vi "111-by.vi"() -> ()   [LabVIEW 2018]
uses:
  Global_Variable/A131258.vi
panel:
  out "9000-10000分贝最小值":string
  out "9000-10000分贝最大值":string
  out "8000-9000分贝最小值":string
  out "8000-9000分贝最大值":string
  out "7000-8000分贝最小值":string
  out "7000-8000分贝最大值":string
  out "6000-7000分贝最小值":string
  out "6000-7000分贝最大值":string
  out "5000-6000分贝最小值":string
  out "5000-6000分贝最大值":string
  out "4000-5000分贝最小值":string
  out "4000-5000分贝最大值":string
  out "3000-4000分贝最小值":string
  out "3000-4000分贝最大值":string
  out "2000-3000分贝最小值":string
  out "2000-3000分贝最大值":string
  out "数组大小":string
  out "1000-2000分贝最小值":string
  out "1000-2000分贝最大值":string
  out "0-1000分贝最小值":string
  out "0-1000分贝最大值":string
  in  "restart averaging (F)":bool
  out "判定结果":bool
  in  "频率":cluster{"f0":dbl, "df":dbl, "magnitude":dbl[]}[](graph)
  out "加速度":cluster{"f0":dbl, "df":dbl, "magnitude":dbl[]}[](graph)
  # "060芯轴总成NVH评价"
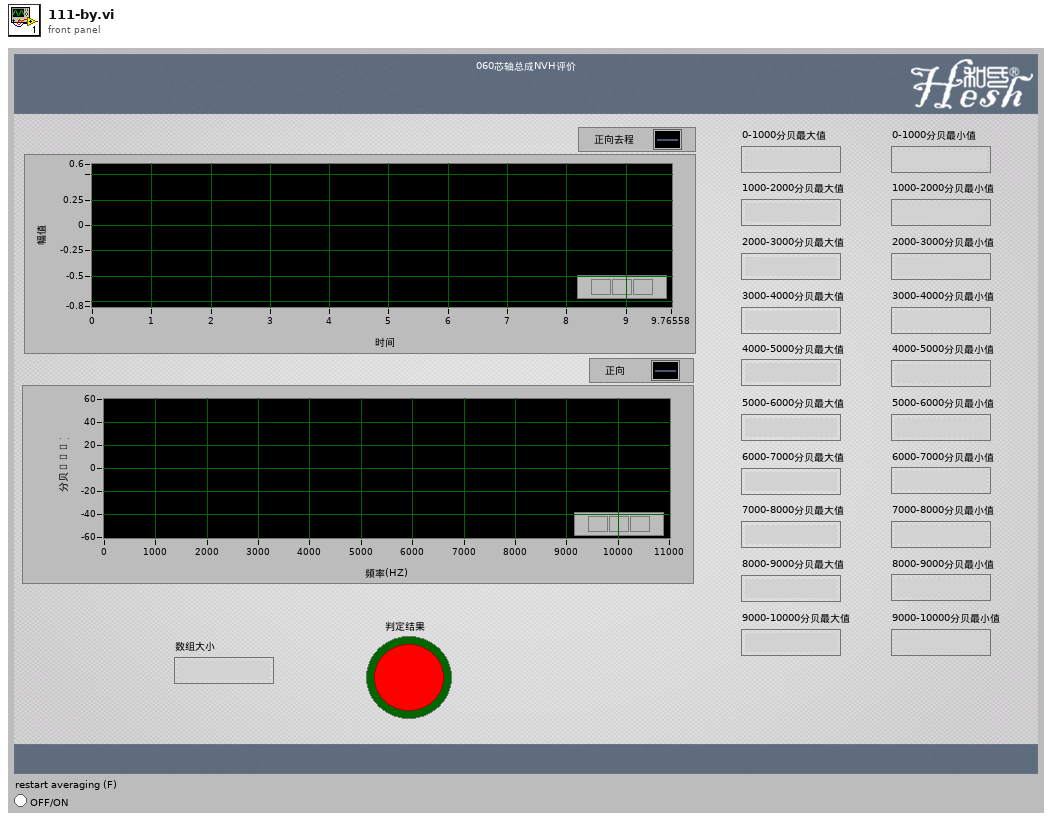
[diagram p1: front panel]
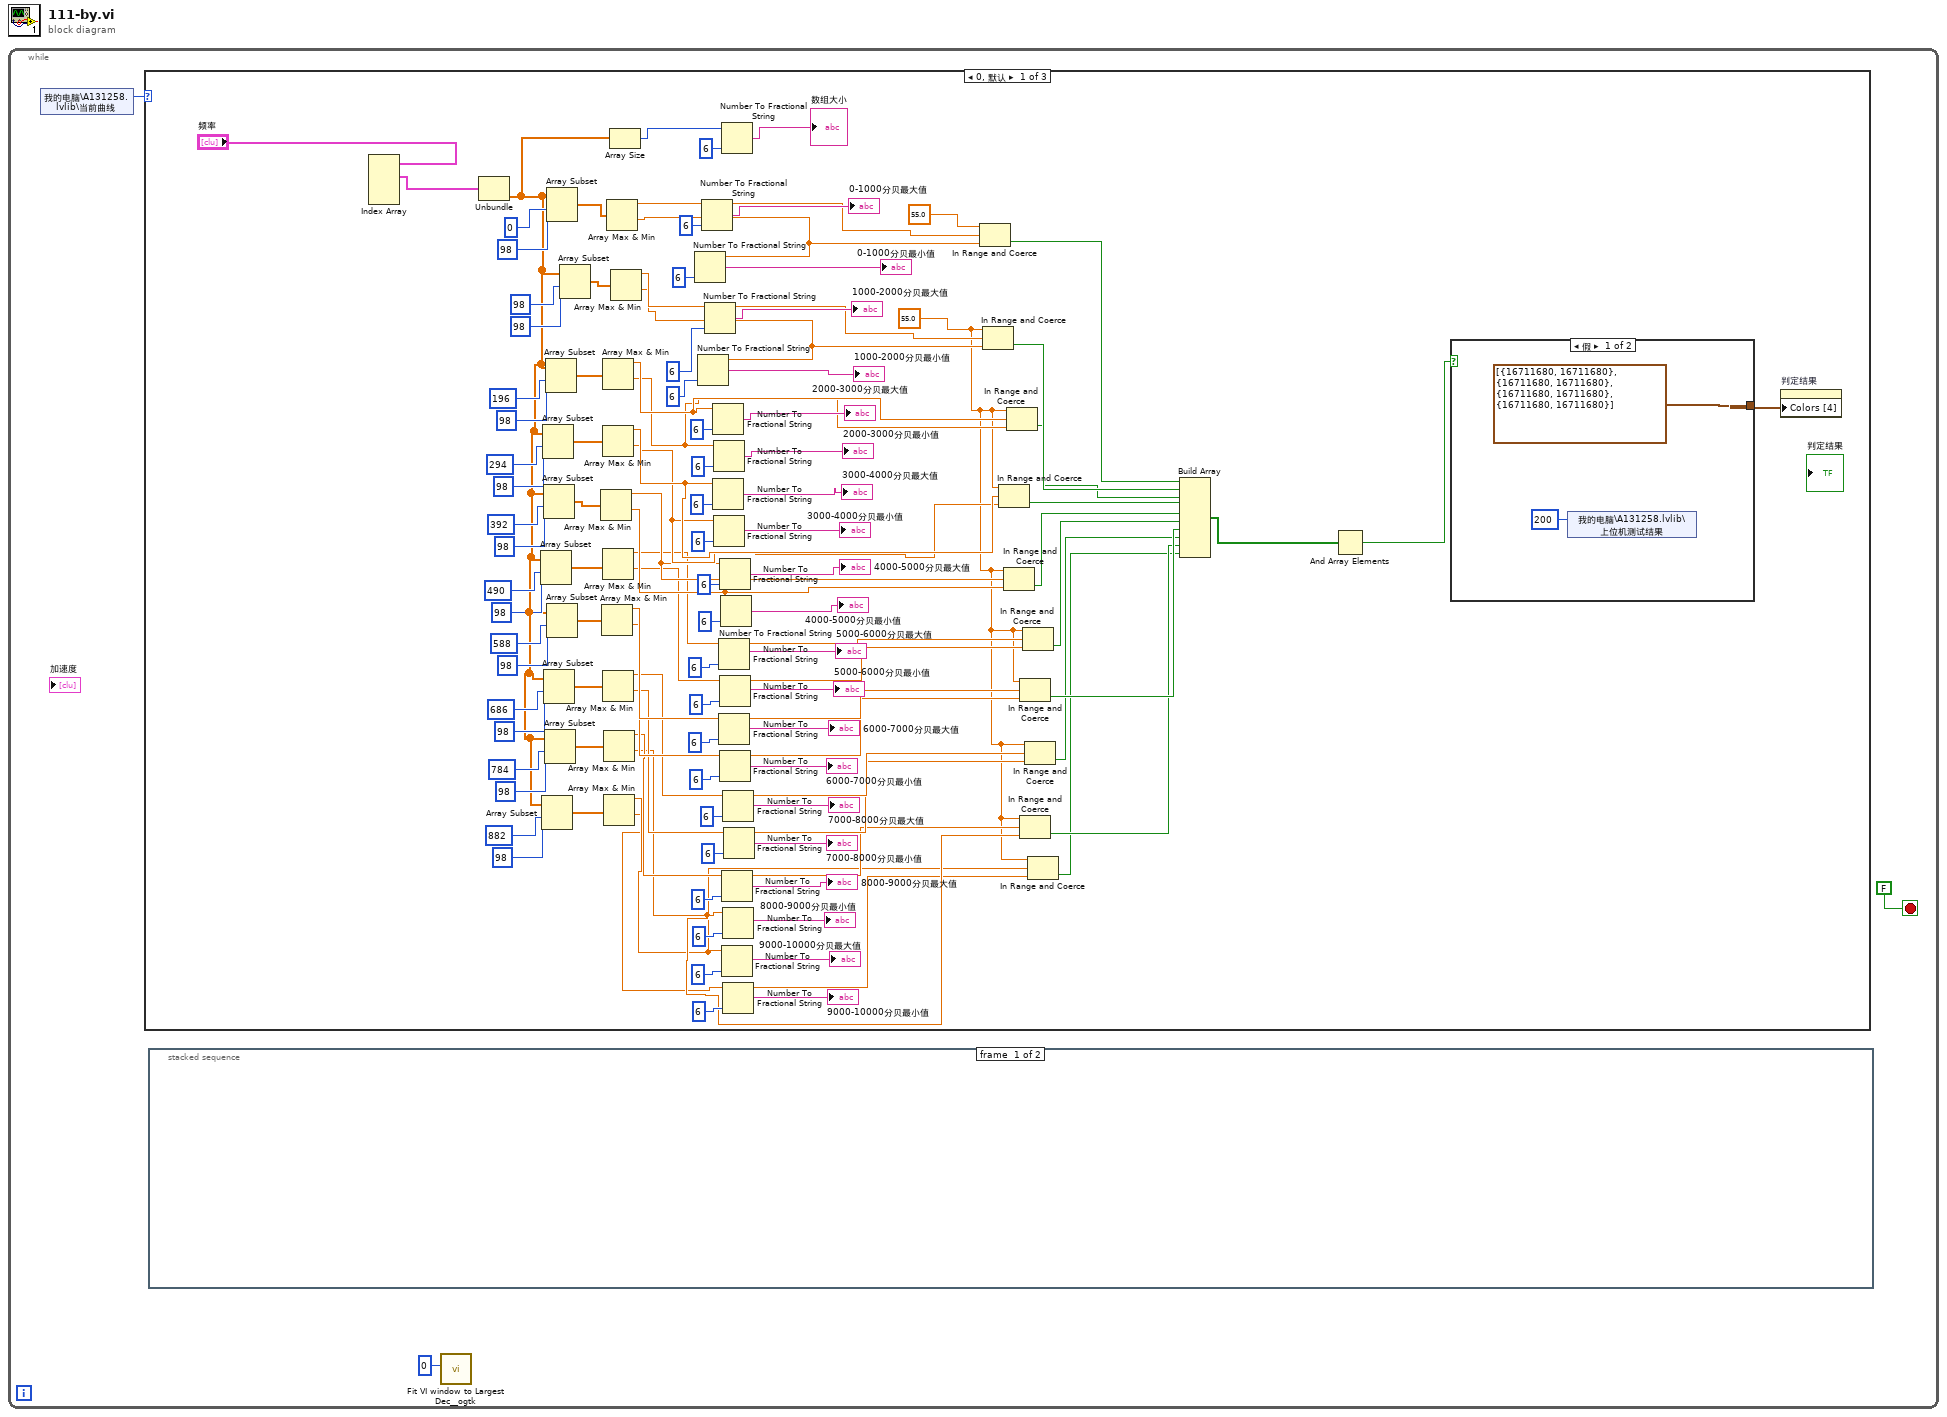
[diagram p0: block diagram]
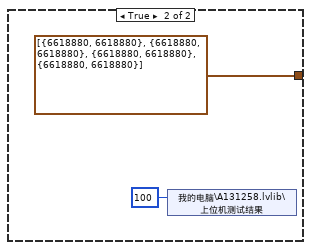
[diagram p3: hidden frame]
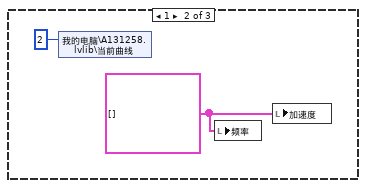
[diagram p4: hidden frame]
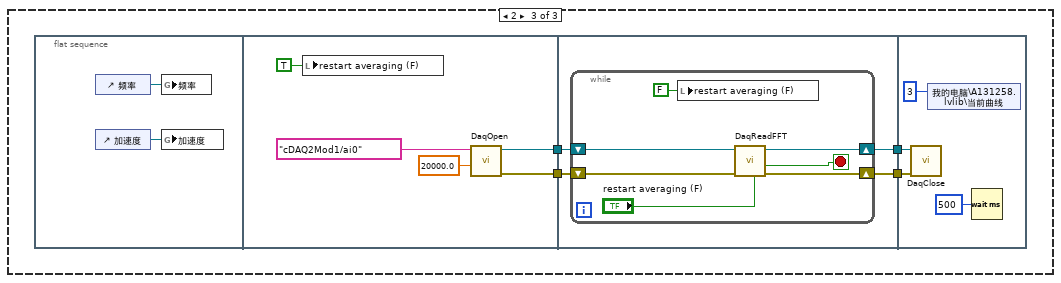
[diagram p5: hidden frame]
diagram:
  n1 = while {
    stop <- FALSE stop-if-true
    n2 = shared-variable "我的电脑\\A131258.lvlib\\当前曲线"() -> (w2:i16)  [unwired: 1 in, 1 out]
    n3 = case shown="0, 默认" w2 {
      frame 0, Default {
        w14 = 55.0 ("x")
        n4 = Index Array(array="频率") -> (element #1=w109:cluster{"f0":dbl, "df":dbl, "magnitude":dbl[]})  [unwired: 4 in, 3 out]
        n5 = Unbundle(w109) -> ("magnitude"=w72:dbl[])  [unwired: 2 out]
        n6 = Array Subset(array=w72, index=490 ("索引"), length=98 ("长度")) -> (w61:dbl[])
        n7 = Array Subset(array=w72, index=882 ("索引"), length=98 ("长度")) -> (w57:dbl[])
        n8 = Array Subset(array=w72, index=294 ("索引"), length=98 ("长度")) -> (w71:dbl[])
        n9 = Array Subset(array=w72, index=392 ("索引"), length=98 ("长度")) -> (w70:dbl[])
        n10 = Array Subset(array=w72, index=686 ("索引"), length=98 ("长度")) -> (w59:dbl[])
        n11 = Array Subset(array=w72, index=784 ("索引"), length=98 ("长度")) -> (w58:dbl[])
        n12 = Array Subset(array=w72, index=196 ("索引"), length=98 ("长度")) -> (w73:dbl[])
        n13 = Array Subset(array=w72, index=0 ("索引"), length=98 ("长度")) -> (w104:dbl[])
        n14 = Array Subset(array=w72, index=588 ("索引"), length=98 ("长度")) -> (w60:dbl[])
        n15 = Array Subset(array=w72, index=98 ("索引"), length=98 ("长度")) -> (w95:dbl[])
        n16 = Array Max & Min(array=w70) -> (max value=w38:dbl, min value=w37:dbl)  [unwired: 2 out]
        n17 = Array Max & Min(array=w60) -> (max value=w34:dbl, min value=w33:dbl)  [unwired: 2 out]
        n18 = Array Max & Min(array=w73) -> (max value=w46:dbl, min value=w45:dbl)  [unwired: 2 out]
        n19 = Array Max & Min(array=w71) -> (max value=w42:dbl, min value=w41:dbl)  [unwired: 2 out]
        n20 = Array Max & Min(array=w61) -> (max value=w36:dbl, min value=w35:dbl)  [unwired: 2 out]
        n21 = Array Max & Min(array=w59) -> (max value=w32:dbl, min value=w31:dbl)  [unwired: 2 out]
        n22 = Array Max & Min(array=w58) -> (max value=w30:dbl, min value=w29:dbl)  [unwired: 2 out]
        n23 = Array Max & Min(array=w57) -> (max value=w28:dbl, min value=w27:dbl)  [unwired: 2 out]
        n24 = Array Max & Min(array=w104) -> (max value=w105:dbl, min value=w108:dbl)  [unwired: 2 out]
        n25 = Array Size(array=w72) -> (size(s)=w91:i32)
        n26 = Array Max & Min(array=w95) -> (max value=w94:dbl, min value=w93:dbl)  [unwired: 2 out]
        n27 = Number To Fractional String(number=w108, precision (6)=i16 6 ("精度(6)")) -> (F-format string=→"0-1000分贝最小值":string)  [unwired: 2 in]
        n28 = Number To Fractional String(number=w93, precision (6)=i16 6 ("精度(6)")) -> (F-format string=→"1000-2000分贝最小值":string)  [unwired: 2 in]
        n29 = Number To Fractional String(number=w105, precision (6)=i16 6 ("精度(6)")) -> (F-format string=→"0-1000分贝最大值":string)  [unwired: 2 in]
        n30 = Number To Fractional String(number=w94, precision (6)=i16 6 ("精度(6)")) -> (F-format string=→"1000-2000分贝最大值":string)  [unwired: 2 in]
        n31 = Number To Fractional String(number=w46, precision (6)=i16 6 ("精度(6)")) -> (F-format string=→"2000-3000分贝最大值":string)  [unwired: 2 in]
        n32 = Number To Fractional String(number=w42, precision (6)=i16 6 ("精度(6)")) -> (F-format string=→"3000-4000分贝最大值":string)  [unwired: 2 in]
        n33 = Number To Fractional String(number=w45, precision (6)=i16 6 ("精度(6)")) -> (F-format string=→"2000-3000分贝最小值":string)  [unwired: 2 in]
        n34 = Number To Fractional String(number=w41, precision (6)=i16 6 ("精度(6)")) -> (F-format string=→"3000-4000分贝最小值":string)  [unwired: 2 in]
        n35 = Number To Fractional String(number=w36, precision (6)=i16 6 ("精度(6)")) -> (F-format string=→"5000-6000分贝最大值":string)  [unwired: 2 in]
        n36 = Number To Fractional String(number=w34, precision (6)=i16 6 ("精度(6)")) -> (F-format string=→"6000-7000分贝最大值":string)  [unwired: 2 in]
        n37 = Number To Fractional String(number=w38, precision (6)=i16 6 ("精度(6)")) -> (F-format string=→"4000-5000分贝最大值":string)  [unwired: 2 in]
        n38 = Number To Fractional String(number=w35, precision (6)=i16 6 ("精度(6)")) -> (F-format string=→"5000-6000分贝最小值":string)  [unwired: 2 in]
        n39 = Number To Fractional String(number=w33, precision (6)=i16 6 ("精度(6)")) -> (F-format string=→"6000-7000分贝最小值":string)  [unwired: 2 in]
        n40 = Number To Fractional String(number=w37, precision (6)=i16 6 ("精度(6)")) -> (F-format string=→"4000-5000分贝最小值":string)  [unwired: 2 in]
        n41 = Number To Fractional String(number=w91, precision (6)=i16 6 ("精度(6)")) -> (F-format string=→"数组大小":string)  [unwired: 2 in]
        n42 = Number To Fractional String(number=w30, precision (6)=i16 6 ("精度(6)")) -> (F-format string=→"8000-9000分贝最大值":string)  [unwired: 2 in]
        n43 = Number To Fractional String(number=w28, precision (6)=i16 6 ("精度(6)")) -> (F-format string=→"9000-10000分贝最大值":string)  [unwired: 2 in]
        n44 = Number To Fractional String(number=w32, precision (6)=i16 6 ("精度(6)")) -> (F-format string=→"7000-8000分贝最大值":string)  [unwired: 2 in]
        n45 = Number To Fractional String(number=w29, precision (6)=i16 6 ("精度(6)")) -> (F-format string=→"8000-9000分贝最小值":string)  [unwired: 2 in]
        n46 = Number To Fractional String(number=w27, precision (6)=i16 6 ("精度(6)")) -> (F-format string=→"9000-10000分贝最小值":string)  [unwired: 2 in]
        n47 = Number To Fractional String(number=w31, precision (6)=i16 6 ("精度(6)")) -> (F-format string=→"7000-8000分贝最小值":string)  [unwired: 2 in]
        n48 = In Range and Coerce(upper limit=55.0 ("x"), x=w105, lower limit=w108) -> (In Range?=w25:bool)  [unwired: 1 out]
        n49 = In Range and Coerce(upper limit=w14, x=w94, lower limit=w93) -> (In Range?=w24:bool)  [unwired: 1 out]
        n50 = In Range and Coerce(upper limit=w14, x=w42, lower limit=w41) -> (In Range?=w22:bool)  [unwired: 1 out]
        n51 = In Range and Coerce(upper limit=w14, x=w38, lower limit=w37) -> (In Range?=w21:bool)  [unwired: 1 out]
        n52 = In Range and Coerce(upper limit=w14, x=w46, lower limit=w45) -> (In Range?=w23:bool)  [unwired: 1 out]
        n53 = In Range and Coerce(upper limit=w14, x=w34, lower limit=w33) -> (In Range?=w19:bool)  [unwired: 1 out]
        n54 = In Range and Coerce(upper limit=w14, x=w30, lower limit=w29) -> (In Range?=w17:bool)  [unwired: 1 out]
        n55 = In Range and Coerce(upper limit=w14, x=w36, lower limit=w35) -> (In Range?=w20:bool)  [unwired: 1 out]
        n56 = In Range and Coerce(upper limit=w14, x=w32, lower limit=w31) -> (In Range?=w18:bool)  [unwired: 1 out]
        n57 = In Range and Coerce(upper limit=w14, x=w28, lower limit=w27) -> (In Range?=w16:bool)  [unwired: 1 out]
        n58 = Build Array(w25, w24, w23, w22, w21, w20, w19, w18, w17, w16) -> (w15:bool[])
        n59 = And Array Elements(Boolean array=w15) -> (logical AND=w26:bool)
        n60 = case shown="假" w26 {
          tunnel: [cluster{u32, u32}[] [{16711680, 16711680}, {16711680, 16711680}, {16711680, 16711680}, {16711680, 16711680}] cluster{u32, u32}[] [{6618880, 6618880}, {6618880, 6618880}, {6618880, 6618880}, {6618880, 6618880}]] -> w107
          frame False {
            n61 = shared-variable "我的电脑\\A131258.lvlib\\上位机测试结果"(i16 200 ("当前曲线")) -> ()  [unwired: 1 in, 1 out]
          }
          frame True {
            n62 = shared-variable "我的电脑\\A131258.lvlib\\上位机测试结果"(i16 100 ("当前曲线")) -> ()  [unwired: 1 in, 1 out]
          }
        }
        n63 = property on="判定结果" class="Bool (严格)"("Colors [4]"=w107) -> ()  [unwired: 2 in, 2 out]
      }
      frame 1 {
        w120 = cluster{"f0":dbl, "df":dbl, "magnitude":dbl[]}[] [] ("添加的数组")
        n64 = shared-variable "我的电脑\\A131258.lvlib\\当前曲线"(i16 2 ("当前曲线")) -> ()  [unwired: 1 in, 1 out]
        n65 = local write "频率"(w120) -> ()
        n66 = local write "加速度"(w120) -> ()
      }
      frame 2 {
        n67 = flat-sequence {
          tunnel: [w130] -> w124
          tunnel: [w129] -> w123
          tunnel: w124 -> [w135]
          tunnel: w123 -> [w134]
          tunnel: [w133] -> w122
          tunnel: [w132] -> w121
          tunnel: w122 -> [w146]
          tunnel: w121 -> [w145]
          frame #0 {
            n68 = control-ref of="频率"() -> (w125:refnum<vi>)
            n69 = control-ref of="加速度"() -> (w126:refnum<vi>)
            n70 = global write "A131258.vi" "频率"(w125) -> ()
            n71 = global write "A131258.vi" "加速度"(w126) -> ()
          }
          frame #1 {
            n72 = local write "restart averaging (F)"(TRUE ("restart averaging (F)")) -> ()
            n73 = call "DaqOpen.vi"("scan rate [S/s]"=20000.0, "physical channels"=tag "cDAQ2Mod1/ai0") -> ("error out"=w129:errorcluster, "task out"=w130:refnum<k21>)  [unwired: 8 in]
          }
          frame #2 {
            n74 = while {
              shift-right: [w139] -> w132
              shift-left: w135 -> [w142]
              shift-right: [w140] -> w133
              shift-left: w134 -> [w141]
              stop <- w138 stop-if-true
              n75 = local write "restart averaging (F)"(FALSE ("restart averaging (F)")) -> ()
              n76 = call "DaqReadFFT.vi"("restart averaging (F)"="restart averaging (F)", "error in"=w141, "task out"=w142) -> ("error out"=w140:errorcluster, "done"=w138:bool, "task out 2"=w139:refnum<k21>)  [unwired: 5 in, 1 out]
            }
          }
          frame #3 {
            n77 = call "DaqClose.vi"("error in"=w146, "task in"=w145) -> ()  [unwired: 9 in, 1 out]
            n78 = shared-variable "我的电脑\\A131258.lvlib\\当前曲线"(i16 3 ("当前曲线")) -> ()  [unwired: 1 in, 1 out]
            n79 = Wait (ms)(milliseconds to wait=u32 500 ("等待时间（毫秒）")) -> ()  [unwired: 1 out]
          }
        }
      }
    }
    n80 = stacked-sequence {
      frame #0 {
      }
      frame #1 {
      }
    }
    n81 = call <userlib>:"Fit VI window to Largest Dec__ogtk.vi"("border spacing (2 px)"=0) -> ()  [unwired: 5 in, 2 out]
  }
